vi "SelectTrajectory.vi"() -> (3 "Robot Action Array":T1)   [LabVIEW 2019]
uses:
  Controls/Trajectory Actions.ctl
  Controls/Enable Actions.ctl
  Controls/Spinner Actions.ctl
  Controls/Ball System Actions.ctl
  Controls/Lift System Actions.ctl
  Controls/Robot Actions Array.ctl
  Controls/Robot Actions.ctl
  Controls/Robot State.ctl
  Controls/Robot Pivot Motion Commands.ctl
  Controls/Pivot Motor Commands.ctl
  Controls/Robot Drive Mode.ctl
  Controls/DriveJoystickData.ctl
  <vilib>/Rock Robotics/Network Tables/NT Read String.vi
  <vilib>/Rock Robotics/Network Tables/NT Write String.vi
panel:
  in  "Tab Control":T12(tab)
  in  "Straight":T13[](array[typedef])=[{"Duration"=0.0, "Front Right Drive Distance (in)"=0.0, "Front Right Steer Angle (deg)"=-90.0, "Front Left Drive Distance (in)"=0.0, "Front Left Steer Angle (deg)"=-90.0, "Rear Left Drive Distance (in)"=0.0, "Rear Left Steer Angle (deg)"=-90.0, "Rear Right Drive Distance (in)"=0.0, "Rear Right Steer Angle (deg)"=-90.0, "Reset Drive Encoder"=FALSE, "Enable Actions"={"Manual Swerve Drive"=FALSE, "Color System"=FALSE, "Ball System"=FALSE, "Lift System"=FALSE}, "SpinnerActions"={"Manual Mode "=FALSE, "Auto rotate n times"=FALSE, "Auto rotate to color\t"=FALSE, "Extend and Retract Arm\t"=FALSE, "Manual Rotation Speed"=0.0}, "Ball System Actions"={"Intake Piston "=FALSE, "Shoot Ball"=FALSE, "Tube up one Increment\t"=FALSE, "Reverse Ball Intake"=FALSE, "Tube Piston"=FALSE, "Enable Manual Tube"=FALSE, "Tube up four Increments"=FALSE, "Manual Tube Velocity"=0.0, "Ball Intake Speed"=0.0, "Color Wheel (Shooter)"=FALSE, "Reverse Shooter"=FALSE}, "Camera Controller"=FALSE, "Lift System Actions"={"Arm Deploy Piston"=FALSE, "Enable Lift Arm"=FALSE, "Enable Climber"=FALSE, "Climber Velocity"=0.0, "Lift Arm Velocity"=0.0}, "AutoFieldSwerveDrive"=FALSE, "Robot Orientation (Deg)"=0.0, "Drive Direction (Deg)"=0.0, "Distance to Drive (in)"=0.0}, {"Duration"=4.0, "Front Right Drive Distance (in)"=0.0, "Front Right Steer Angle (deg)"=-90.0, "Front Left Drive Distance (in)"=0.0, "Front Left Steer Angle (deg)"=-90.0, "Rear Left Drive Distance (in)"=0.0, "Rear Left Steer Angle (deg)"=-90.0, "Rear Right Drive Distance (in)"=0.0, "Rear Right Steer Angle (deg)"=-90.0, "Reset Drive Encoder"=FALSE, "Enable Actions"={"Manual Swerve Drive"=TRUE, "Color System"=FALSE, "Ball System"=TRUE, "Lift System"=FALSE}, "SpinnerActions"={"Manual Mode "=FALSE, "Auto rotate n times"=FALSE, "Auto rotate to color\t"=FALSE, "Extend and Retract Arm\t"=FALSE, "Manual Rotation Speed"=0.0}, "Ball System Actions"={"Intake Piston "=FALSE, "Shoot Ball"=TRUE, "Tube up one Increment\t"=FALSE, "Reverse Ball Intake"=FALSE, "Tube Piston"=FALSE, "Enable Manual Tube"=FALSE, "Tube up four Increments"=FALSE, "Manual Tube Velocity"=0.0, "Ball Intake Speed"=0.0, "Color Wheel (Shooter)"=FALSE, "Reverse Shooter"=FALSE}, "Camera Controller"=FALSE, "Lift System Actions"={"Arm Deploy Piston"=FALSE, "Enable Lift Arm"=FALSE, "Enable Climber"=FALSE, "Climber Velocity"=0.0, "Lift Arm Velocity"=0.0}, "AutoFieldSwerveDrive"=FALSE, "Robot Orientation (Deg)"=0.0, "Drive Direction (Deg)"=0.0, "Distance to Drive (in)"=0.0}, {"Duration"=6.0, "Front Right Drive Distance (in)"=0.0, "Front Right Steer Angle (deg)"=-90.0, "Front Left Drive Distance (in)"=0.0, "Front Left Steer Angle (deg)"=-90.0, "Rear Left Drive Distance (in)"=0.0, "Rear Left Steer Angle (deg)"=-90.0, "Rear Right Drive Distance (in)"=0.0, "Rear Right Steer Angle (deg)"=-90.0, "Reset Drive Encoder"=FALSE, "Enable Actions"={"Manual Swerve Drive"=TRUE, "Color System"=FALSE, "Ball System"=TRUE, "Lift System"=FALSE}, "SpinnerActions"={"Manual Mode "=FALSE, "Auto rotate n times"=FALSE, "Auto rotate to color\t"=FALSE, "Extend and Retract Arm\t"=FALSE, "Manual Rotation Speed"=0.0}, "Ball System Actions"={"Intake Piston "=FALSE, "Shoot Ball"=TRUE, "Tube up one Increment\t"=FALSE, "Reverse Ball Intake"=FALSE, "Tube Piston"=FALSE, "Enable Manual Tube"=TRUE, "Tube up four Increments"=FALSE, "Manual Tube Velocity"=-1.0, "Ball Intake Speed"=0.0, "Color Wheel (Shooter)"=FALSE, "Reverse Shooter"=FALSE}, "Camera Controller"=FALSE, "Lift System Actions"={"Arm Deploy Piston"=FALSE, "Enable Lift Arm"=FALSE, "Enable Climber"=FALSE, "Climber Velocity"=0.0, "Lift Arm Velocity"=0.0}, "AutoFieldSwerveDrive"=FALSE, "Robot Orientation (Deg)"=0.0, "Drive Direction (Deg)"=0.0, "Distance to Drive (in)"=0.0}, {"Duration"=4.0, "Front Right Drive Distance (in)"=-45.0, "Front Right Steer Angle (deg)"=-90.0, "Front Left Drive Distance (in)"=-45.0, "Front Left Steer Angle (deg)"=-90.0, "Rear Left Drive Distance (in)"=-45.0, "Rear Left Steer Angle (deg)"=-90.0, "Rear Right Drive Distance (in)"=-45.0, "Rear Right Steer Angle (deg)"=-90.0, "Reset Drive Encoder"=FALSE, "Enable Actions"={"Manual Swerve Drive"=TRUE, "Color System"=FALSE, "Ball System"=TRUE, "Lift System"=FALSE}, "SpinnerActions"={"Manual Mode "=FALSE, "Auto rotate n times"=FALSE, "Auto rotate to color\t"=FALSE, "Extend and Retract Arm\t"=FALSE, "Manual Rotation Speed"=0.0}, "Ball System Actions"={"Intake Piston "=FALSE, "Shoot Ball"=FALSE, "Tube up one Increment\t"=FALSE, "Reverse Ball Intake"=FALSE, "Tube Piston"=FALSE, "Enable Manual Tube"=FALSE, "Tube up four Increments"=FALSE, "Manual Tube Velocity"=-1.0, "Ball Intake Speed"=0.0, "Color Wheel (Shooter)"=FALSE, "Reverse Shooter"=FALSE}, "Camera Controller"=FALSE, "Lift System Actions"={"Arm Deploy Piston"=FALSE, "Enable Lift Arm"=FALSE, "Enable Climber"=FALSE, "Climber Velocity"=0.0, "Lift Arm Velocity"=0.0}, "AutoFieldSwerveDrive"=FALSE, "Robot Orientation (Deg)"=0.0, "Drive Direction (Deg)"=0.0, "Distance to Drive (in)"=0.0}, {"Duration"=0.1, "Front Right Drive Distance (in)"=-45.0, "Front Right Steer Angle (deg)"=-90.0, "Front Left Drive Distance (in)"=-45.0, "Front Left Steer Angle (deg)"=-90.0, "Rear Left Drive Distance (in)"=-45.0, "Rear Left Steer Angle (deg)"=-90.0, "Rear Right Drive Distance (in)"=-45.0, "Rear Right Steer Angle (deg)"=-90.0, "Reset Drive Encoder"=TRUE, "Enable Actions"={"Manual Swerve Drive"=TRUE, "Color System"=FALSE, "Ball System"=TRUE, "Lift System"=FALSE}, "SpinnerActions"={"Manual Mode "=FALSE, "Auto rotate n times"=FALSE, "Auto rotate to color\t"=FALSE, "Extend and Retract Arm\t"=FALSE, "Manual Rotation Speed"=0.0}, "Ball System Actions"={"Intake Piston "=FALSE, "Shoot Ball"=FALSE, "Tube up one Increment\t"=FALSE, "Reverse Ball Intake"=FALSE, "Tube Piston"=FALSE, "Enable Manual Tube"=FALSE, "Tube up four Increments"=FALSE, "Manual Tube Velocity"=0.0, "Ball Intake Speed"=0.0, "Color Wheel (Shooter)"=FALSE, "Reverse Shooter"=FALSE}, "Camera Controller"=FALSE, "Lift System Actions"={"Arm Deploy Piston"=FALSE, "Enable Lift Arm"=FALSE, "Enable Climber"=FALSE, "Climber Velocity"=0.0, "Lift Arm Velocity"=0.0}, "AutoFieldSwerveDrive"=FALSE, "Robot Orientation (Deg)"=0.0, "Drive Direction (Deg)"=0.0, "Distance to Drive (in)"=0.0}]
  in  "Camera":T13[](array[typedef])=[{"Duration"=0.0, "Front Right Drive Distance (in)"=0.0, "Front Right Steer Angle (deg)"=0.0, "Front Left Drive Distance (in)"=0.0, "Front Left Steer Angle (deg)"=0.0, "Rear Left Drive Distance (in)"=0.0, "Rear Left Steer Angle (deg)"=0.0, "Rear Right Drive Distance (in)"=0.0, "Rear Right Steer Angle (deg)"=0.0, "Reset Drive Encoder"=FALSE, "Enable Actions"={"Manual Swerve Drive"=FALSE, "Color System"=FALSE, "Ball System"=FALSE, "Lift System"=FALSE}, "SpinnerActions"={"Manual Mode "=FALSE, "Auto rotate n times"=FALSE, "Auto rotate to color\t"=FALSE, "Extend and Retract Arm\t"=FALSE, "Manual Rotation Speed"=0.0}, "Ball System Actions"={"Intake Piston "=FALSE, "Shoot Ball"=FALSE, "Tube up one Increment\t"=FALSE, "Reverse Ball Intake"=FALSE, "Tube Piston"=FALSE, "Enable Manual Tube"=FALSE, "Tube up four Increments"=FALSE, "Manual Tube Velocity"=0.0, "Ball Intake Speed"=0.0, "Color Wheel (Shooter)"=FALSE, "Reverse Shooter"=FALSE}, "Camera Controller"=FALSE, "Lift System Actions"={"Arm Deploy Piston"=FALSE, "Enable Lift Arm"=FALSE, "Enable Climber"=FALSE, "Climber Velocity"=0.0, "Lift Arm Velocity"=0.0}, "AutoFieldSwerveDrive"=FALSE, "Robot Orientation (Deg)"=0.0, "Drive Direction (Deg)"=0.0, "Distance to Drive (in)"=0.0}, {"Duration"=4.0, "Front Right Drive Distance (in)"=0.0, "Front Right Steer Angle (deg)"=0.0, "Front Left Drive Distance (in)"=0.0, "Front Left Steer Angle (deg)"=0.0, "Rear Left Drive Distance (in)"=0.0, "Rear Left Steer Angle (deg)"=0.0, "Rear Right Drive Distance (in)"=0.0, "Rear Right Steer Angle (deg)"=0.0, "Reset Drive Encoder"=FALSE, "Enable Actions"={"Manual Swerve Drive"=FALSE, "Color System"=FALSE, "Ball System"=TRUE, "Lift System"=FALSE}, "SpinnerActions"={"Manual Mode "=FALSE, "Auto rotate n times"=FALSE, "Auto rotate to color\t"=FALSE, "Extend and Retract Arm\t"=FALSE, "Manual Rotation Speed"=0.0}, "Ball System Actions"={"Intake Piston "=FALSE, "Shoot Ball"=TRUE, "Tube up one Increment\t"=FALSE, "Reverse Ball Intake"=FALSE, "Tube Piston"=FALSE, "Enable Manual Tube"=FALSE, "Tube up four Increments"=FALSE, "Manual Tube Velocity"=0.0, "Ball Intake Speed"=0.0, "Color Wheel (Shooter)"=FALSE, "Reverse Shooter"=FALSE}, "Camera Controller"=TRUE, "Lift System Actions"={"Arm Deploy Piston"=FALSE, "Enable Lift Arm"=FALSE, "Enable Climber"=FALSE, "Climber Velocity"=0.0, "Lift Arm Velocity"=0.0}, "AutoFieldSwerveDrive"=FALSE, "Robot Orientation (Deg)"=0.0, "Drive Direction (Deg)"=0.0, "Distance to Drive (in)"=0.0}, {"Duration"=6.0, "Front Right Drive Distance (in)"=0.0, "Front Right Steer Angle (deg)"=0.0, "Front Left Drive Distance (in)"=0.0, "Front Left Steer Angle (deg)"=0.0, "Rear Left Drive Distance (in)"=0.0, "Rear Left Steer Angle (deg)"=0.0, "Rear Right Drive Distance (in)"=0.0, "Rear Right Steer Angle (deg)"=0.0, "Reset Drive Encoder"=FALSE, "Enable Actions"={"Manual Swerve Drive"=FALSE, "Color System"=FALSE, "Ball System"=TRUE, "Lift System"=FALSE}, "SpinnerActions"={"Manual Mode "=FALSE, "Auto rotate n times"=FALSE, "Auto rotate to color\t"=FALSE, "Extend and Retract Arm\t"=FALSE, "Manual Rotation Speed"=0.0}, "Ball System Actions"={"Intake Piston "=FALSE, "Shoot Ball"=TRUE, "Tube up one Increment\t"=FALSE, "Reverse Ball Intake"=FALSE, "Tube Piston"=FALSE, "Enable Manual Tube"=TRUE, "Tube up four Increments"=FALSE, "Manual Tube Velocity"=-1.0, "Ball Intake Speed"=0.0, "Color Wheel (Shooter)"=FALSE, "Reverse Shooter"=FALSE}, "Camera Controller"=FALSE, "Lift System Actions"={"Arm Deploy Piston"=FALSE, "Enable Lift Arm"=FALSE, "Enable Climber"=FALSE, "Climber Velocity"=0.0, "Lift Arm Velocity"=0.0}, "AutoFieldSwerveDrive"=FALSE, "Robot Orientation (Deg)"=0.0, "Drive Direction (Deg)"=0.0, "Distance to Drive (in)"=0.0}, {"Duration"=4.0, "Front Right Drive Distance (in)"=-33.0, "Front Right Steer Angle (deg)"=0.0, "Front Left Drive Distance (in)"=-33.0, "Front Left Steer Angle (deg)"=0.0, "Rear Left Drive Distance (in)"=-33.0, "Rear Left Steer Angle (deg)"=0.0, "Rear Right Drive Distance (in)"=-33.0, "Rear Right Steer Angle (deg)"=0.0, "Reset Drive Encoder"=FALSE, "Enable Actions"={"Manual Swerve Drive"=TRUE, "Color System"=FALSE, "Ball System"=FALSE, "Lift System"=FALSE}, "SpinnerActions"={"Manual Mode "=FALSE, "Auto rotate n times"=FALSE, "Auto rotate to color\t"=FALSE, "Extend and Retract Arm\t"=FALSE, "Manual Rotation Speed"=0.0}, "Ball System Actions"={"Intake Piston "=FALSE, "Shoot Ball"=FALSE, "Tube up one Increment\t"=FALSE, "Reverse Ball Intake"=FALSE, "Tube Piston"=FALSE, "Enable Manual Tube"=FALSE, "Tube up four Increments"=FALSE, "Manual Tube Velocity"=0.0, "Ball Intake Speed"=0.0, "Color Wheel (Shooter)"=FALSE, "Reverse Shooter"=FALSE}, "Camera Controller"=FALSE, "Lift System Actions"={"Arm Deploy Piston"=FALSE, "Enable Lift Arm"=FALSE, "Enable Climber"=FALSE, "Climber Velocity"=0.0, "Lift Arm Velocity"=0.0}, "AutoFieldSwerveDrive"=FALSE, "Robot Orientation (Deg)"=0.0, "Drive Direction (Deg)"=0.0, "Distance to Drive (in)"=0.0}]
  in  "Set up Robot":T13[](array[typedef])=[{"Duration"=0.0, "Front Right Drive Distance (in)"=0.0, "Front Right Steer Angle (deg)"=0.0, "Front Left Drive Distance (in)"=0.0, "Front Left Steer Angle (deg)"=0.0, "Rear Left Drive Distance (in)"=0.0, "Rear Left Steer Angle (deg)"=0.0, "Rear Right Drive Distance (in)"=0.0, "Rear Right Steer Angle (deg)"=0.0, "Reset Drive Encoder"=FALSE, "Enable Actions"={"Manual Swerve Drive"=FALSE, "Color System"=FALSE, "Ball System"=FALSE, "Lift System"=FALSE}, "SpinnerActions"={"Manual Mode "=FALSE, "Auto rotate n times"=FALSE, "Auto rotate to color\t"=FALSE, "Extend and Retract Arm\t"=FALSE, "Manual Rotation Speed"=0.0}, "Ball System Actions"={"Intake Piston "=FALSE, "Shoot Ball"=FALSE, "Tube up one Increment\t"=FALSE, "Reverse Ball Intake"=FALSE, "Tube Piston"=FALSE, "Enable Manual Tube"=FALSE, "Tube up four Increments"=FALSE, "Manual Tube Velocity"=0.0, "Ball Intake Speed"=0.0, "Color Wheel (Shooter)"=FALSE, "Reverse Shooter"=FALSE}, "Camera Controller"=FALSE, "Lift System Actions"={"Arm Deploy Piston"=FALSE, "Enable Lift Arm"=FALSE, "Enable Climber"=FALSE, "Climber Velocity"=0.0, "Lift Arm Velocity"=0.0}, "AutoFieldSwerveDrive"=FALSE, "Robot Orientation (Deg)"=0.0, "Drive Direction (Deg)"=0.0, "Distance to Drive (in)"=0.0}, {"Duration"=4.0, "Front Right Drive Distance (in)"=0.0, "Front Right Steer Angle (deg)"=-90.0, "Front Left Drive Distance (in)"=0.0, "Front Left Steer Angle (deg)"=-90.0, "Rear Left Drive Distance (in)"=0.0, "Rear Left Steer Angle (deg)"=-90.0, "Rear Right Drive Distance (in)"=0.0, "Rear Right Steer Angle (deg)"=-90.0, "Reset Drive Encoder"=FALSE, "Enable Actions"={"Manual Swerve Drive"=FALSE, "Color System"=FALSE, "Ball System"=FALSE, "Lift System"=FALSE}, "SpinnerActions"={"Manual Mode "=FALSE, "Auto rotate n times"=FALSE, "Auto rotate to color\t"=FALSE, "Extend and Retract Arm\t"=FALSE, "Manual Rotation Speed"=0.0}, "Ball System Actions"={"Intake Piston "=FALSE, "Shoot Ball"=FALSE, "Tube up one Increment\t"=FALSE, "Reverse Ball Intake"=FALSE, "Tube Piston"=FALSE, "Enable Manual Tube"=FALSE, "Tube up four Increments"=FALSE, "Manual Tube Velocity"=0.0, "Ball Intake Speed"=0.0, "Color Wheel (Shooter)"=FALSE, "Reverse Shooter"=FALSE}, "Camera Controller"=FALSE, "Lift System Actions"={"Arm Deploy Piston"=FALSE, "Enable Lift Arm"=FALSE, "Enable Climber"=FALSE, "Climber Velocity"=0.0, "Lift Arm Velocity"=0.0}, "AutoFieldSwerveDrive"=FALSE, "Robot Orientation (Deg)"=0.0, "Drive Direction (Deg)"=0.0, "Distance to Drive (in)"=0.0}, {"Duration"=0.0, "Front Right Drive Distance (in)"=0.0, "Front Right Steer Angle (deg)"=0.0, "Front Left Drive Distance (in)"=0.0, "Front Left Steer Angle (deg)"=0.0, "Rear Left Drive Distance (in)"=0.0, "Rear Left Steer Angle (deg)"=0.0, "Rear Right Drive Distance (in)"=0.0, "Rear Right Steer Angle (deg)"=0.0, "Reset Drive Encoder"=FALSE, "Enable Actions"={"Manual Swerve Drive"=FALSE, "Color System"=FALSE, "Ball System"=FALSE, "Lift System"=FALSE}, "SpinnerActions"={"Manual Mode "=FALSE, "Auto rotate n times"=FALSE, "Auto rotate to color\t"=FALSE, "Extend and Retract Arm\t"=FALSE, "Manual Rotation Speed"=0.0}, "Ball System Actions"={"Intake Piston "=FALSE, "Shoot Ball"=FALSE, "Tube up one Increment\t"=FALSE, "Reverse Ball Intake"=FALSE, "Tube Piston"=FALSE, "Enable Manual Tube"=FALSE, "Tube up four Increments"=FALSE, "Manual Tube Velocity"=0.0, "Ball Intake Speed"=0.0, "Color Wheel (Shooter)"=FALSE, "Reverse Shooter"=FALSE}, "Camera Controller"=FALSE, "Lift System Actions"={"Arm Deploy Piston"=FALSE, "Enable Lift Arm"=FALSE, "Enable Climber"=FALSE, "Climber Velocity"=0.0, "Lift Arm Velocity"=0.0}, "AutoFieldSwerveDrive"=FALSE, "Robot Orientation (Deg)"=0.0, "Drive Direction (Deg)"=0.0, "Distance to Drive (in)"=0.0}, {"Duration"=0.0, "Front Right Drive Distance (in)"=0.0, "Front Right Steer Angle (deg)"=0.0, "Front Left Drive Distance (in)"=0.0, "Front Left Steer Angle (deg)"=0.0, "Rear Left Drive Distance (in)"=0.0, "Rear Left Steer Angle (deg)"=0.0, "Rear Right Drive Distance (in)"=0.0, "Rear Right Steer Angle (deg)"=0.0, "Reset Drive Encoder"=FALSE, "Enable Actions"={"Manual Swerve Drive"=FALSE, "Color System"=FALSE, "Ball System"=FALSE, "Lift System"=FALSE}, "SpinnerActions"={"Manual Mode "=FALSE, "Auto rotate n times"=FALSE, "Auto rotate to color\t"=FALSE, "Extend and Retract Arm\t"=FALSE, "Manual Rotation Speed"=0.0}, "Ball System Actions"={"Intake Piston "=FALSE, "Shoot Ball"=FALSE, "Tube up one Increment\t"=FALSE, "Reverse Ball Intake"=FALSE, "Tube Piston"=FALSE, "Enable Manual Tube"=FALSE, "Tube up four Increments"=FALSE, "Manual Tube Velocity"=0.0, "Ball Intake Speed"=0.0, "Color Wheel (Shooter)"=FALSE, "Reverse Shooter"=FALSE}, "Camera Controller"=FALSE, "Lift System Actions"={"Arm Deploy Piston"=FALSE, "Enable Lift Arm"=FALSE, "Enable Climber"=FALSE, "Climber Velocity"=0.0, "Lift Arm Velocity"=0.0}, "AutoFieldSwerveDrive"=FALSE, "Robot Orientation (Deg)"=0.0, "Drive Direction (Deg)"=0.0, "Distance to Drive (in)"=0.0}]
  # "Note that the first element in the trajectory is only the starting state and the duration is ignored."
  # "MAKE CURRENT VALUE DEFAULT BEFORE SAVING!!!!"
  # "Positive is a turn to the right\ni.e. Drive Direction of 90 is move right\nDrive Direction of 180 is move backwards\nRobot Orientation of 90 is a turn to right"
  # "Positive is a turn to the right\ni.e. Drive Direction of 90 is move right\nDrive Direction of 180 is move backwards\nRobot Orientation of 90 is a turn to right"
  # "Positive is a turn to the right\ni.e. Drive Direction of 90 is move right\nDrive Direction of 180 is move backwards\nRobot Orientation of 90 is a turn to right"
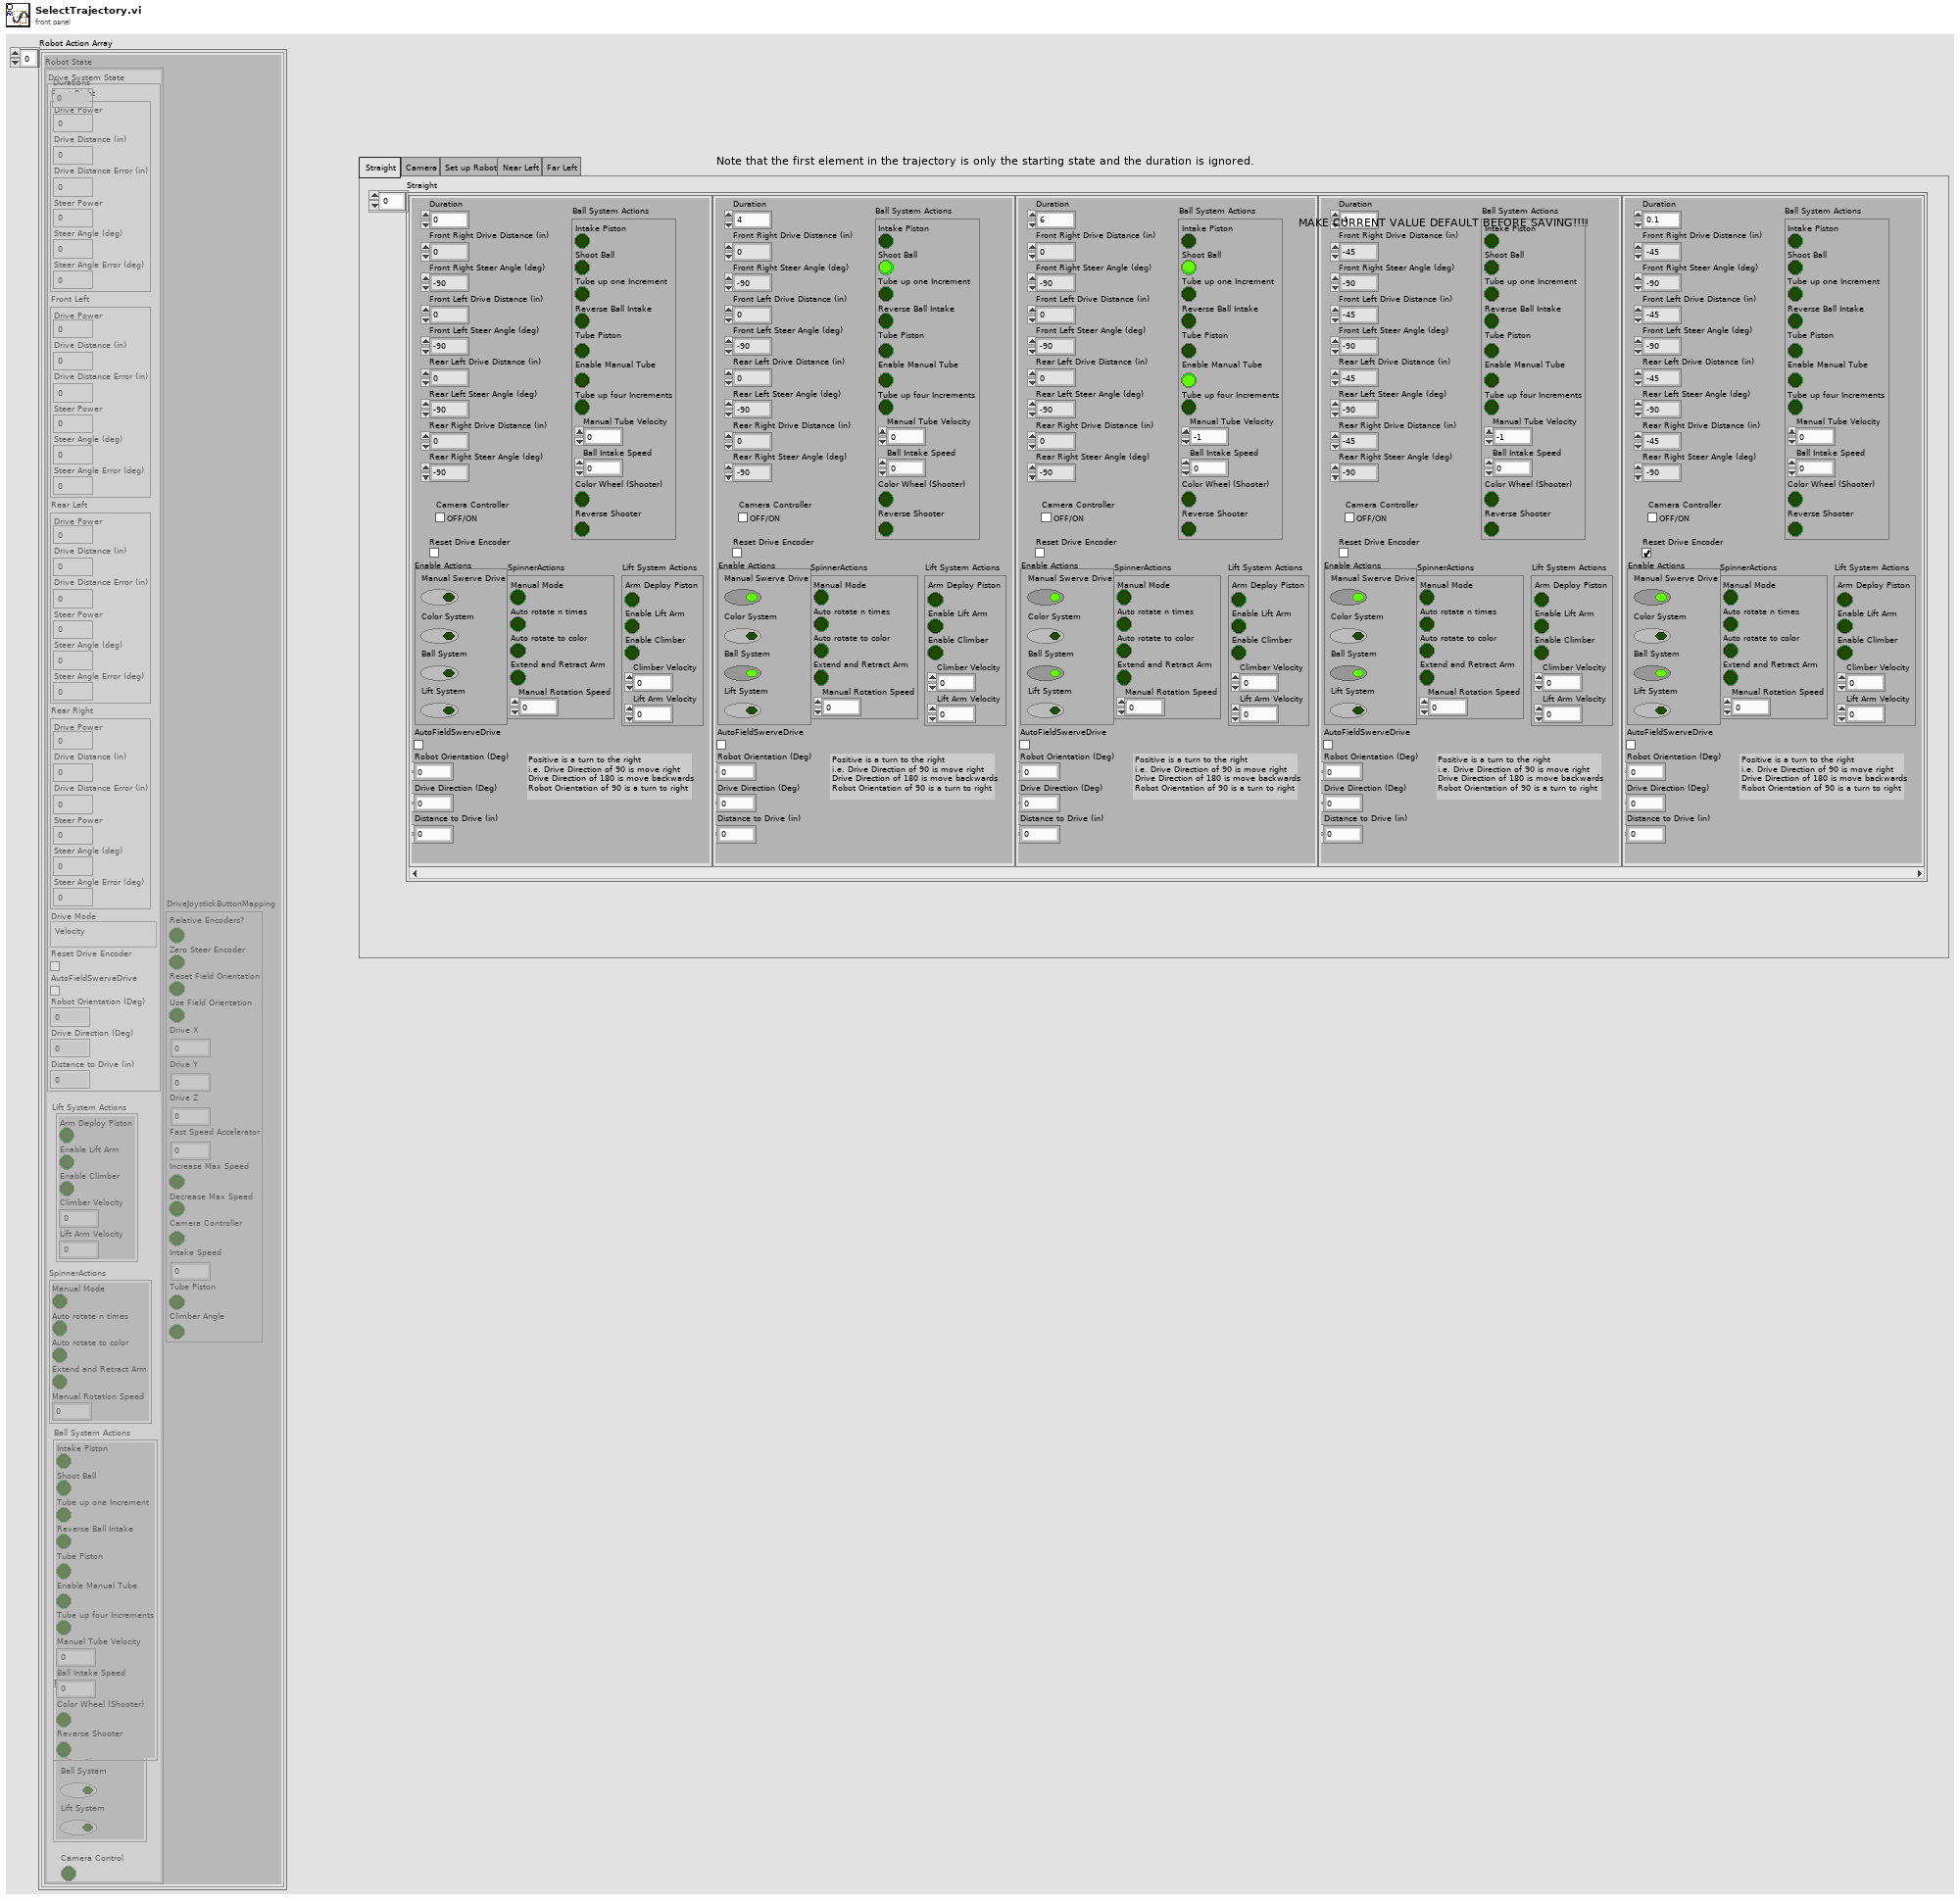
[diagram p1: front panel]
types:
  T1 = typedef "Robot Actions Array.ctl" = T2[]
  T2 = typedef "Robot Actions.ctl" = cluster{"Durations":dbl, "Robot State":T3, "DriveJoystickButtonMapping":T11}
  T3 = typedef "Robot State.ctl" = cluster{"Drive System State":T4, "Enable Actions":T7, "Lift System Actions":T8, "SpinnerActions":T9, "Ball System Actions":T10, "Camera Control":bool}
  T4 = typedef "Robot Pivot Motion Commands.ctl" = cluster{"Front Right":T5, "Front Left":T5, "Rear Left":T5, "Rear Right":T5, "Drive Mode":T6, "Reset Drive Encoder":bool, "AutoFieldSwerveDrive":bool, "Robot Orientation (Deg)":dbl, "Drive Direction (Deg)":dbl, "Distance to Drive (in)":dbl}
  T5 = typedef "Pivot Motor Commands.ctl" = cluster{"Drive Power":dbl, "Drive Distance (in)":dbl, "Drive Distance Error (in)":dbl, "Steer Power":dbl, "Steer Angle (deg)":dbl, "Steer Angle Error (deg)":dbl}
  T6 = typedef "Robot Drive Mode.ctl" = enum16{"Velocity", "Distance"}
  T7 = typedef "Enable Actions.ctl" = cluster{"Manual Swerve Drive":bool, "Color System":bool, "Ball System":bool, "Lift System":bool}
  T8 = typedef "Lift System Actions.ctl" = cluster{"Arm Deploy Piston":bool, "Enable Lift Arm":bool, "Enable Climber":bool, "Climber Velocity":dbl, "Lift Arm Velocity":dbl}
  T9 = typedef "Spinner Actions.ctl" = cluster{"Manual Mode ":bool, "Auto rotate n times":bool, "Auto rotate to color\t":bool, "Extend and Retract Arm\t":bool, "Manual Rotation Speed":dbl}
  T10 = typedef "Ball System Actions.ctl" = cluster{"Intake Piston ":bool, "Shoot Ball":bool, "Tube up one Increment\t":bool, "Reverse Ball Intake":bool, "Tube Piston":bool, "Enable Manual Tube":bool, "Tube up four Increments":bool, "Manual Tube Velocity":dbl, "Ball Intake Speed":dbl, "Color Wheel (Shooter)":bool, "Reverse Shooter":bool}
  T11 = typedef "DriveJoystickData.ctl" = cluster{"Relative Encoders?":bool, "Zero Steer Encoder":bool, "Reset Field Orientation":bool, "Use Field Orientation":bool, "Drive X":dbl, "Drive Y":dbl, "Drive Z":dbl, "Fast Speed Accelerator":dbl, "Increase Max Speed":bool, "Decrease Max Speed":bool, "Camera Controller":bool, "Intake Speed":dbl, "Tube Piston":bool, "Climber Angle":bool}
  T12 = enum32{"Straight ", "Camera", "Set up Robot", "Near Left", "Far Left"}
  T13 = typedef "Trajectory Actions.ctl" = cluster{"Duration":dbl, "Front Right Drive Distance (in)":dbl, "Front Right Steer Angle (deg)":dbl, "Front Left Drive Distance (in)":dbl, "Front Left Steer Angle (deg)":dbl, "Rear Left Drive Distance (in)":dbl, "Rear Left Steer Angle (deg)":dbl, "Rear Right Drive Distance (in)":dbl, "Rear Right Steer Angle (deg)":dbl, "Reset Drive Encoder":bool, "Enable Actions":T7, "SpinnerActions":T9, "Ball System Actions":T10, "Camera Controller":bool, "Lift System Actions":T8, "AutoFieldSwerveDrive":bool, "Robot Orientation (Deg)":dbl, "Drive Direction (Deg)":dbl, "Distance to Drive (in)":dbl}
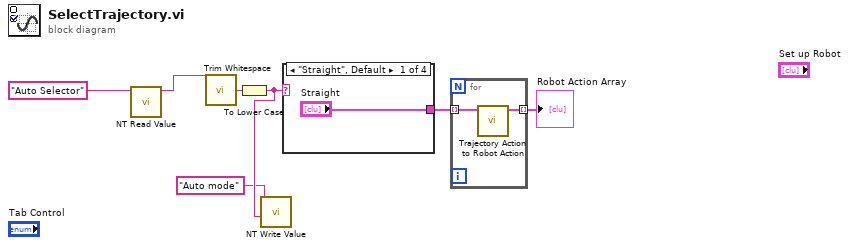
[diagram p0: block diagram]
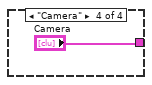
[diagram p4: hidden frame]
diagram:
  n1 = call-poly <vilib>:"NT Read Value.vi"("Name"="Auto Selector") -> ("String"=w1:string)  [unwired: 9 in, 1 out]
  n2 = call <vilib>:"Trim Whitespace.vi"("string"=w1) -> ("trimmed string"=w6:string)  [unwired: 1 in]
  n3 = To Lower Case(string=w6) -> (all lower case string=w3:string)
  n4 = call-poly <vilib>:"NT Write Value.vi"("String"=w3, "Name"="Auto mode") -> ()  [unwired: 9 in, 1 out]
  n5 = case shown="\"Straight\", Default" w3 {
    tunnel: ["Straight" _ _ "Camera"] -> w5
    frame "Straight", Default {
    }
    frame "Near Left" {
    }
    frame "Far Left" {
    }
    frame "Camera" {
    }
  }
  n6 = for {
    tunnel: [w11] -> w4 mode=indexing
    tunnel: w5 -> [w10] mode=indexing
    n7 = call "Trajectory Action to Robot Action.vi"("Trajectory Action"=w10) -> ("Robot Action"=w11:T2)  [unwired: 10 in]
  }
  "Robot Action Array" <- w4
